vi "New Dispay Settings.vi"(8 "error in (no error)":errorcluster, 10 "Display settings":T1, 11 "IMAQ Display in":refnum<class "HIJ Vision Display.lvclass">) -> (0 "error out":errorcluster, 3 "IMAQ Display out":refnum<class "HIJ Vision Display.lvclass">)   [LabVIEW 2020, in "HIJ Vision Display.lvlib" / "HIJ Vision Display.lvclass"]
uses:
  HIJ Vision Display.lvclass
  C:/Program Files (x86)/National Instruments/LabVIEW 2020/vi.lib/ActorFramework/Actor/Actor.lvclass
  DisplaySettings.ctl
  Analyze/Analyze Parameter/Analyze Parameter Target Point/Target Point.lvclass
  C:/POLARIS Programme/POLARIS-AS-3-Cams/Submodules/HIJ Vision/Analyze/Analyze Parameter/Analyze Parameter Base/Analyze Parameter Base.lvclass
  Analyze/Analyze Parameter/Analyze Parameter Calibration/Analyze Parameter Calibration.lvclass
  HIJ Vision Display.lvclass/HIJ Vision Display.ctl
  Analyze/Analyze Parameter/Analyze Parameter Calibration/Analyze Parameter Calibration.lvclass/Analyze Parameter Calibration.ctl
  Analyze/Analyze Parameter/Analyze Parameter Target Point/Target Point.lvclass/Target Point.ctl
  <vilib>/ActorFramework/Actor/Actor.lvclass/Actor.ctl
  <vilib>/ActorFramework/Message Enqueuer/Message Enqueuer.lvclass/Message Enqueuer.ctl
  Analyze/Analyze Actor/Analyze Actor Messages/Set Analyze Parameter Msg/Set Analyze Parameter Msg.lvclass/Set Analyze Parameter Msg.ctl
  Analyze/Analyze Parameter/Analyze Parameter Target Point/Write target point.vi
  Analyze/Analyze Parameter/Analyze Parameter Calibration/Write Calibration.vi
  <vilib>/ActorFramework/Message Enqueuer/Init from Existing Queue.vi
  <vilib>/ActorFramework/Message Enqueuer/Enqueue.vi
  Analyze/Analyze Actor/Analyze Actor Messages/Set Analyze Parameter Msg/Set Analyze Parameter Msg.lvclass
  C:/Program Files (x86)/National Instruments/LabVIEW 2020/vi.lib/ActorFramework/Message/Message.lvclass
  HIJ Vision Display Messages/Evaluate with new Params Msg/Evaluate with new Params Msg.lvclass
  <vilib>/ActorFramework/Message Priority Queue/Priority Enqueue.vi
  <vilib>/ActorFramework/Message Enqueuer/Message Enqueuer.lvclass
  <vilib>/ActorFramework/Actor/Actor.lvclass
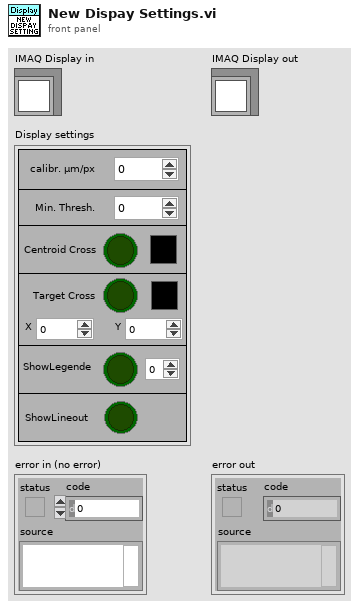
[diagram p1: front panel]
types:
  T1 = typedef "HIJ Vision Display.lvlib/HIJ Vision Display.lvclass/DisplaySettings.ctl" = cluster{"Min. Thresh.":sgl, "X":dbl, "Y":dbl, "ShowLineout":bool, "ScaleParts":i32, "ShowLegende":bool, "Target Cross":bool, "Centroid Cross":bool, "Target color":u32, "Centroid color":u32, "calibr. µm/px":sgl[unit]}
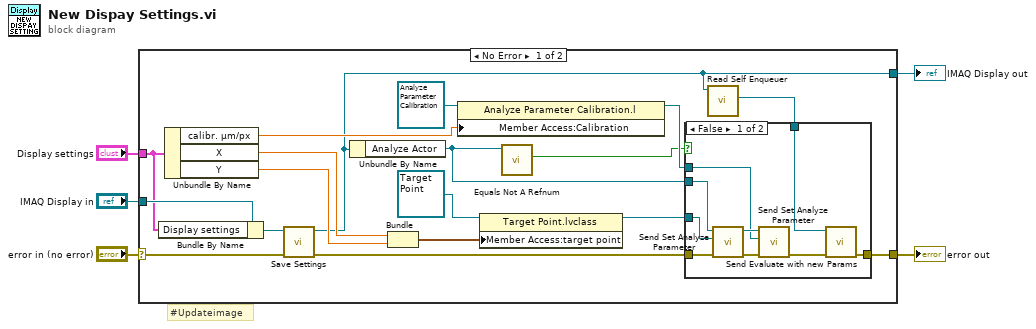
[diagram p0: block diagram]
diagram:
  # "#Updateimage"
  n1 = case shown="No Error" "error in (no error)" {
    selector: "error in (no error)" -> [w21 w35]
    tunnel: [w11 w35] -> w4
    tunnel: [w7 w34] -> w2
    tunnel: "IMAQ Display in" -> [w23 w34]
    tunnel: "Display settings" -> [w19 _]
    frame No Error {
      n2 = Bundle By Name(cluster=w23, "Display settings"=w19) -> (w22:refnum<class "HIJ Vision Display.lvclass">)
      n3 = Unbundle By Name(w19) -> ("calibr. µm/px"=w8:sgl[unit], "X"=w18:dbl, "Y"=w17:dbl)
      n4 = call-dynamic "Save Settings.vi"("error in (no error)"=w21, "IMAQ Display in"=w22) -> ("error out"=w12:errorcluster, "IMAQ Display out"=w7:refnum<class "HIJ Vision Display.lvclass">)  [unwired: 8 in]
      n5 = Unbundle By Name(w7) -> ("Analyze Actor"=w10:refnum<class "Message Enqueuer.lvclass">)
      n6 = Bundle("X"=w18, "Y"=w17) -> (w16:cluster{"X":dbl, "Y":dbl})  [unwired: 1 in]
      n7 = property class="Analyze Parameter Calibration.l"(reference=refnum<class "Analyze Parameter Calibration.lvclass"> refnum ("Analyze Parameter Calibration.lvclass"), "Member Access:Calibration"=w8) -> (reference out=w13:refnum<class "Analyze Parameter Calibration.lvclass">)  [unwired: 1 in, 1 out]
      n8 = property class="Target Point.lvclass"(reference=refnum<class "Target Point.lvclass"> refnum ("Target Point.lvclass"), "Member Access:target point"=w16) -> (reference out=w15:refnum<class "Target Point.lvclass">)  [unwired: 1 in, 1 out]
      n9 = call <vilib>:"Equals Not A Refnum.vi"("Message Enqueuer"=w10) -> ("Not a refnum?"=w9:bool)  [unwired: 10 in]
      n10 = call <vilib>:"Read Self Enqueuer.vi"("Actor"=w7) -> ("Self Enqueuer"=w6:refnum<class "Message Enqueuer.lvclass">)  [unwired: 10 in]
      n11 = case shown="False" w9 {
        tunnel: w10 -> [w32 _]
        tunnel: w15 -> [w29 _]
        tunnel: w13 -> [w28 _]
        tunnel: w12 -> [w27 w33]
        tunnel: [w25 w33] -> w11
        tunnel: w6 -> [w24 _]
        frame False {
          n12 = call "Send Set Analyze Parameter.vi"("error in (no error)"=w27, "Analyze Parameter"=w29, "Message Enqueuer"=w32) -> ("error out"=w31:errorcluster, "Message Enqueuer out"=w30:refnum<class "Message Enqueuer.lvclass">)  [unwired: 7 in]
          n13 = call "Send Set Analyze Parameter.vi"("error in (no error)"=w31, "Analyze Parameter"=w28, "Message Enqueuer"=w30) -> ("error out"=w26:errorcluster)  [unwired: 7 in, 1 out]
          n14 = call "Send Evaluate with new Params.vi"("error in (no error)"=w26, "Message Enqueuer"=w24) -> ("error out"=w25:errorcluster)  [unwired: 8 in, 1 out]
        }
        frame True {
        }
      }
    }
    frame Error {
    }
  }
  "error out" <- w4
  "IMAQ Display out" <- w2
